vi "子界面-图像预处理.vi"(11 "原图":T2(plugin-control)) -> (3 "处理后":T2(plugin-control))   [LabVIEW 2018]
uses:
  <vilib>/vision/NI_Vision_Development_Module.lvlib
panel:
  in  "Operation":T1(ring)
  in  "返回":bool
  in  "确认":bool
  in  "结构元素":i32[][](array[numeric])=[[1, 1, 1], [1, 1, 1], [1, 1, 1]]
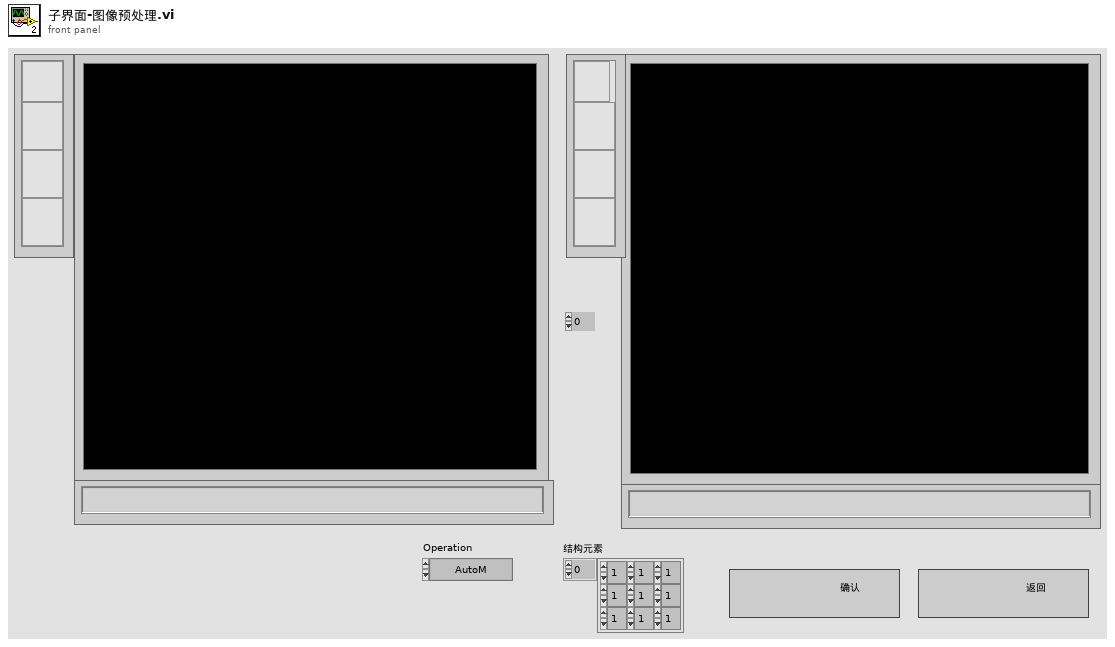
[diagram p1: front panel]
types:
  T1 = enum32{"AutoM", "Close", "Dilate", "Erode", "Gradient", "Gradient in", "Gradient out", "HitMiss", "Open", "PClose", "POpen", "Thick", "Thin"}
  T2 = typedef "IMAQ Image.ctl" = refnum<image>
  T3 = typedef "Image Type" = u32
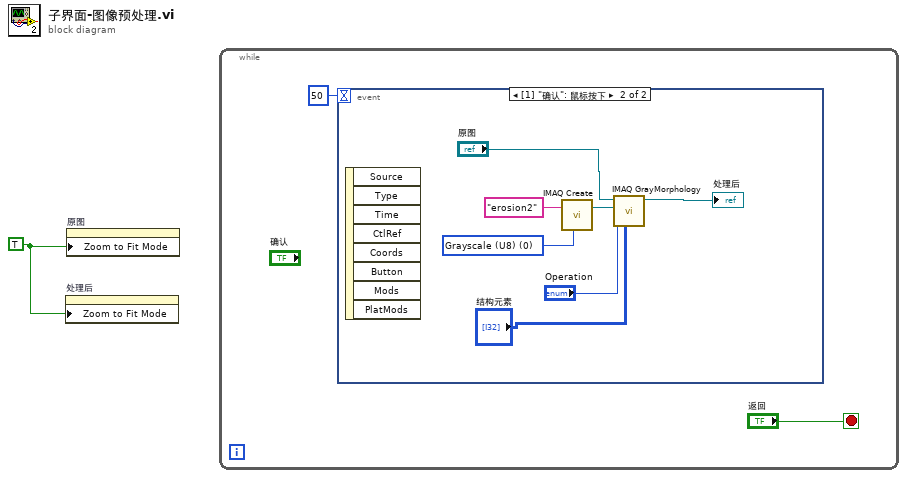
[diagram p0: block diagram]
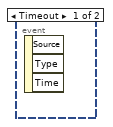
[diagram p2: hidden frame]
diagram:
  w1 = TRUE ("Zoom to Fit Mode")
  n1 = property on="处理后" class="ImageControl"("Zoom to Fit Mode"=w1) -> ()  [unwired: 2 in, 2 out]
  n2 = property on="原图" class="ImageControl"("Zoom to Fit Mode"=w1) -> ()  [unwired: 2 in, 2 out]
  n3 = while {
    stop <- "返回" stop-if-true
    n4 = event shown="[1] \"确认\": 鼠标按下" {
      selector: _ -> [_ _]
      dyn-events: _ -> [_ _]
      timeout: 50 -> [_ _]
      event Timeout {
        n5 = event-data() -> ()  [unwired: 1 in, 3 out]
      }
      event "确认": Mouse Down {
        w7 = T3 0 items=["Grayscale (U8)", "Grayscale (I16)", "Grayscale (SGL)", "Complex (CSG)", "RGB (U32)", "HSL (U32)", "RGB (U64)", "Grayscale (U16)"] ("Image Type")
        n6 = event-data() -> ()  [unwired: 1 in, 8 out]
        n7 = call "IMAQ Create"("Image Name"="erosion2", "Image Type"=w7) -> ("New Image"=w9:T2)  [unwired: 3 in, 1 out]
        n8 = call "IMAQ GrayMorphology"("Structuring Element"="结构元素", "Operation"="Operation", "Image Dst"=w9, "Image Src"="原图") -> ("Image Dst Out"=→"处理后":T2)  [unwired: 6 in, 1 out]
      }
    }
  }
